vi "Convert_All_subs.vi"(3 "Shift in":string[](array[string]), 4 "Saved Vis paths in":string[](array[string]), 5 "Top level VI Name":string, 6 "VI path":path) -> (0 "Shift out":string[](array[string]), 1 "Saved Vis paths Out":string[](array[string]), 2 "Exec.State":T1(ring))   [LabVIEW 2010]
panel:
  in  "stop":bool
  out "Current array size":i32
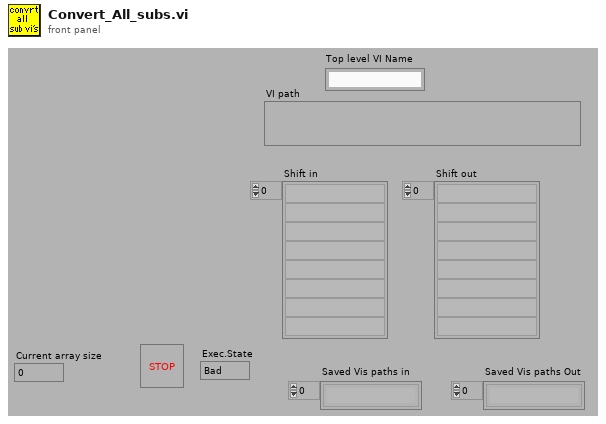
[diagram p1: front panel]
types:
  T1 = enum32{"Bad", "Idle", "Run top level", "Running"}
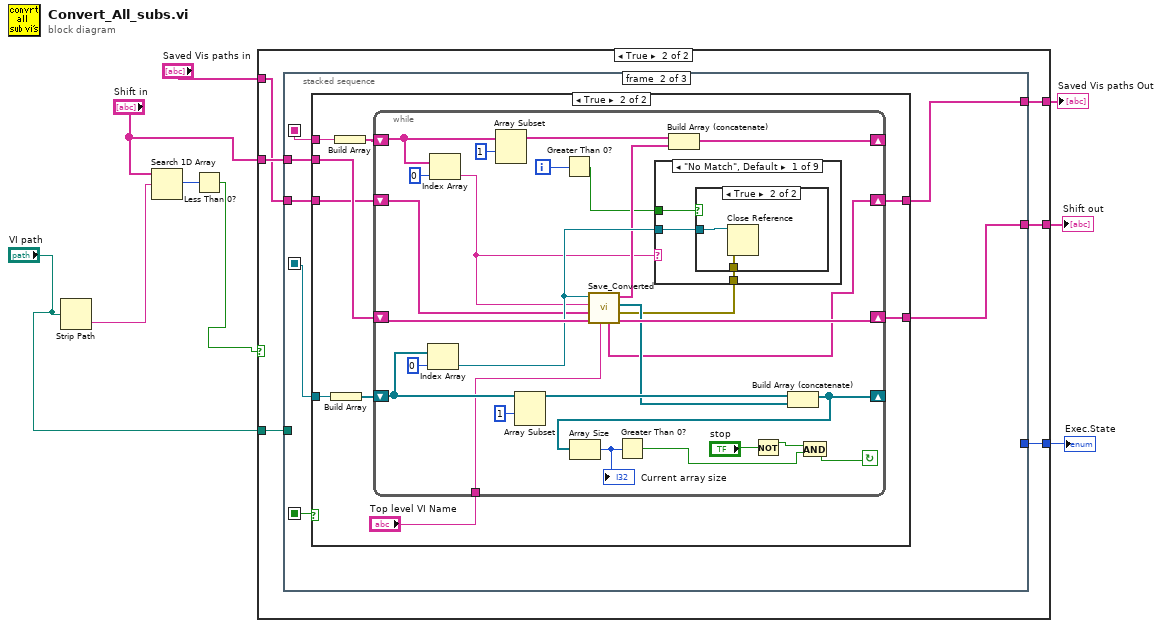
[diagram p0: block diagram]
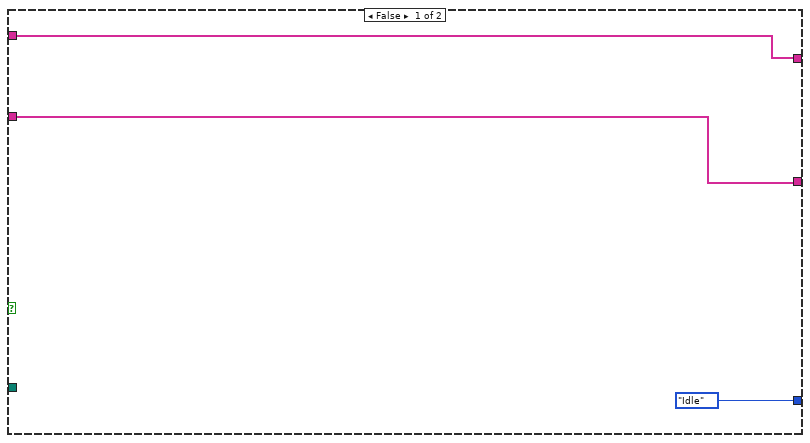
[diagram p2: hidden frame]
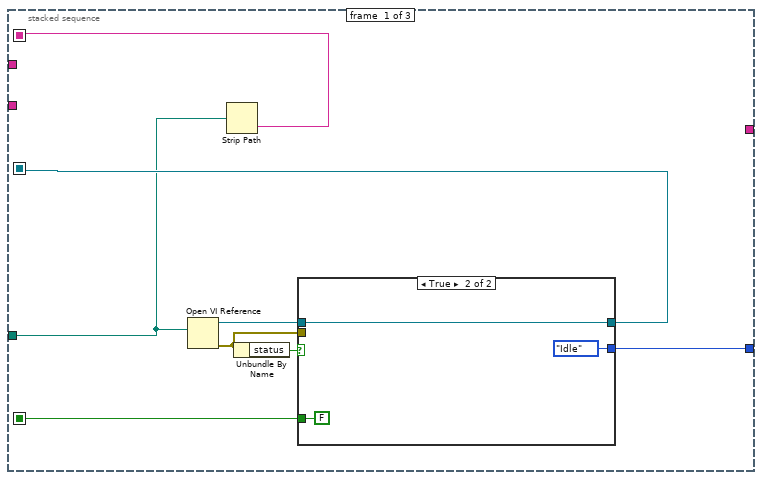
[diagram p3: hidden frame]
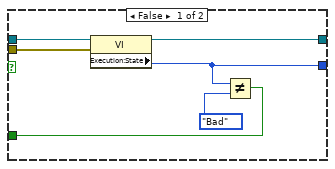
[diagram p4: hidden frame]
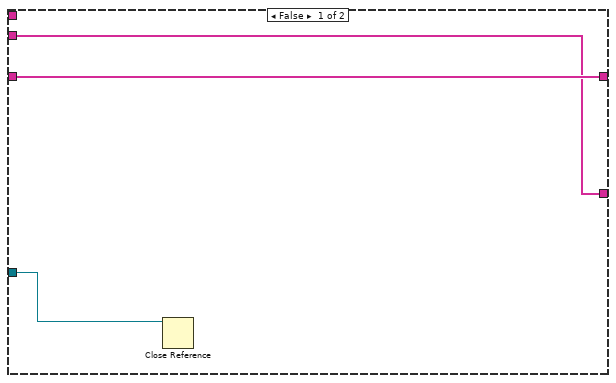
[diagram p5: hidden frame]
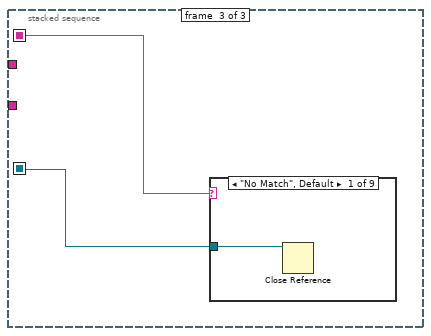
[diagram p15: hidden frame]
diagram:
  n1 = Strip Path(path="VI path") -> (name=w4:string)  [unwired: 1 out]
  n2 = Search 1D Array(1D array="Shift in", element=w4) -> (index of element=w3:i32)  [unwired: 1 out]
  n3 = Less Than 0?(x=w3) -> (x < 0?=w1:bool)
  n4 = case shown="True" w1 {
    tunnel: "VI path" -> [_ w18]
    tunnel: "Shift in" -> [w12 w17]
    tunnel: [w12 w16] -> w9
    tunnel: [T1."Idle" ("Exec.State") w15] -> w8
    tunnel: "Saved Vis paths in" -> [w10 w14]
    tunnel: [w10 w13] -> w6
    frame False {
    }
    frame True {
      n5 = stacked-sequence {
        seq-local: [w26 _ _] -> [_ w42 w87]
        seq-local: [w24 _ _] -> [_ w39 w88]
        seq-local: [w22 _ _] -> [_ w38 _]
        tunnel: w18 -> [w25 _ _]
        tunnel: w17 -> [_ w41 _]
        tunnel: [_ w40 _] -> w16
        tunnel: [w23 _ _] -> w15
        tunnel: w14 -> [_ w37 _]
        tunnel: [_ w36 _] -> w13
        frame #0 {
          n6 = Open VI Reference(vi path=w25) -> (vi reference=w21:refnum<vi>, error out=w20:errorcluster)  [unwired: 1 in, 4 out]
          n7 = Strip Path(path=w25) -> (name=w24:string)  [unwired: 1 out]
          n8 = Unbundle By Name(w20) -> ("status"=w19:bool)
          n9 = case shown="True" w19 {
            tunnel: [w32 w33] -> w26
            tunnel: w20 -> [w31 _]
            tunnel: [w30 T1."Idle" ("Exec.State")] -> w23
            tunnel: [w28 FALSE] -> w22
            tunnel: w21 -> [w27 w33]
            frame False {
              n10 = property class="VI"(reference=w27, error in=w31) -> (reference out=w32:refnum<vi>, "Execution:State"=w30:T1)  [unwired: 1 out]
              n11 = Not Equal?(x=w30, y=T1."Bad" ("Exec.State")) -> (x != y?=w28:bool)
            }
            frame True {
            }
          }
        }
        frame #1 {
          n12 = case shown="True" w38 {
            tunnel: w42 -> [w43 w54]
            tunnel: w41 -> [w44 w51]
            tunnel: [w44 w50] -> w40
            tunnel: w37 -> [w45 w49]
            tunnel: [w45 w48] -> w36
            tunnel: w39 -> [_ w47]
            frame False {
              n13 = Close Reference(reference=w43) -> ()  [unwired: 1 in, 1 out]
            }
            frame True {
              n14 = Build Array(w54) -> (w53:refnum<vi>[])
              n15 = Build Array(w47) -> (w52:string[])
              n16 = while {
                shift-left: w49 -> [w63]
                shift-right: [w62] -> w48
                shift-left: w52 -> [w59]
                shift-right: [w64] -> _
                shift-left: w51 -> [w72]
                shift-right: [w71] -> w50
                shift-left: w53 -> [w79]
                shift-right: [w69] -> _
                tunnel: "Top level VI Name" -> [w55]
                i -> [w61]
                stop <- w77 continue-if-true
                n17 = Index Array(array=w79, index=0) -> (element=w67:refnum<vi>)
                n18 = Index Array(array=w59, index=0) -> (element=w57:string)
                n19 = Array Subset(array=w59, index=1) -> (w65:string[])  [unwired: 1 in]
                n20 = Array Subset(array=w79, index=1) -> (w73:refnum<vi>[])  [unwired: 1 in]
                n21 = Greater Than 0?(x=w61) -> (x > 0?=w56:bool)
                n22 = call "Save_Converted.vi"("Top level VI Name"=w55, "Vi's already saved in"=w72, "Saved Vis paths in"=w63, "VI to save"=w57, "vi reference"=w67) -> ("Vi's already saved out"=w71:string[], "Error IO"=w68:errorcluster, "vi references to save"=w70:refnum<vi>[], "Vi's that need saving"=w58:string[], "Saved Vis paths Out"=w62:string[])  [unwired: 2 out]
                n23 = case shown="\"No Match\", Default" w57 {
                  tunnel: w68 -> [w84 _ _ _ _ _ _ _ _]
                  tunnel: w67 -> [w83 _ _ _ _ _ _ _ _]
                  tunnel: w56 -> [w82 _ _ _ _ _ _ _ _]
                  frame "No Match", Default {
                    n24 = case shown="True" w82 {
                      tunnel: w83 -> [_ w86]
                      tunnel: w84 -> [_ w85]
                      frame False {
                      }
                      frame True {
                        n25 = Close Reference(reference=w86, error in (no error)=w85) -> ()  [unwired: 1 out]
                      }
                    }
                  }
                  frame "Do ADAM channel" {
                  }
                  frame "Measurement" {
                  }
                  frame "Calibration" {
                  }
                  frame "Read Ch data file" {
                  }
                  frame "Write Ch data file" {
                  }
                  frame "Set Traverse Position" {
                  }
                  frame "Set Source" {
                  }
                  frame "Multiport Serial Tx_Rx_tl.vi" {
                  }
                }
                n26 = Build Array (concatenate)(w65, w58) -> (w64:string[])
                n27 = Not(x="stop") -> (.not. x?=w78:bool)
                n28 = Build Array (concatenate)(w73, w70) -> (w69:refnum<vi>[])
                n29 = Array Size(array=w69) -> (size(s)=w76:i32)
                "Current array size" <- w76
                n30 = Greater Than 0?(x=w76) -> (x > 0?=w75:bool)
                n31 = And(x=w78, y=w75) -> (x .and. y?=w77:bool)
              }
            }
          }
        }
        frame #2 {
          n32 = case shown="\"No Match\", Default" w88 {
            tunnel: w87 -> [w89 _ _ _ _ _ _ _ _]
            frame "No Match", Default {
              n33 = Close Reference(reference=w89) -> ()  [unwired: 1 in, 1 out]
            }
            frame "Do ADAM channel" {
            }
            frame "Set Traverse Position" {
            }
            frame "Set Source" {
            }
            frame "Multiport Serial Tx_Rx_tl.vi" {
            }
            frame "Measurement" {
            }
            frame "Write Ch data file" {
            }
            frame "Calibration" {
            }
            frame "Read Ch data file" {
            }
          }
        }
      }
    }
  }
  "Shift out" <- w9
  "Exec.State" <- w8
  "Saved Vis paths Out" <- w6
